vi "Weibull Moments.vi"(9 "b":dbl=3.0, 10 "a":dbl=1.0) -> (0 "error":i32, 2 "variance":dbl=1.0, 3 "mean":dbl)   [LabVIEW 2020, in "NI_Gmath.lvlib"]
doc: "Returns the expected mean and variance of the random variate X, where X describes the selected distribution type. You must manually select the polymorphic instance to use."
uses:
  <vilib>/gmath/NI_Gmath.lvlib
  <vilib>/gmath/statdist.llb/st_error_code.ctl
  <vilib>/gmath/SpecialFunctions.llb/Gamma Function.vi
panel:
  # "Weibull Moments"
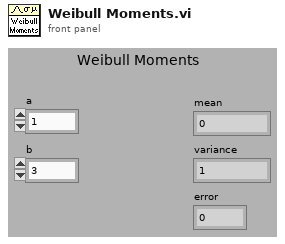
[diagram p1: front panel]
types:
  T1 = typedef "NI_Gmath.lvlib/st_error_code.ctl" = i32
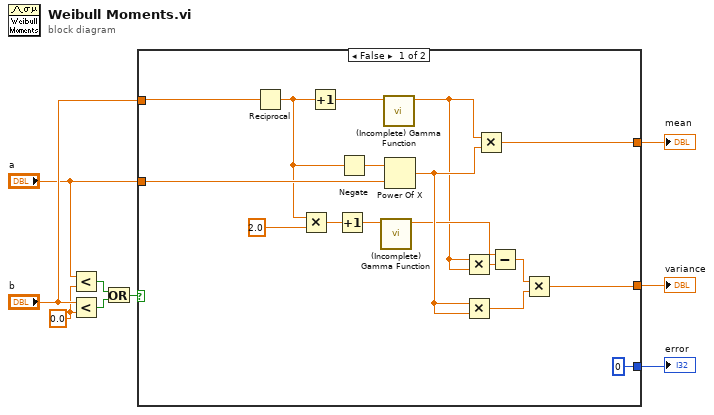
[diagram p0: block diagram]
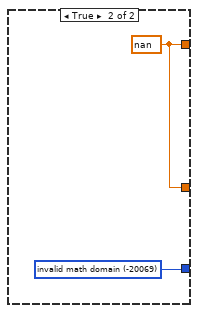
[diagram p2: hidden frame]
diagram:
  w6 = 0.0 ("y")
  n1 = Less?(x="a", y=w6) -> (x < y?=w2:bool)
  n2 = Less?(x="b", y=w6) -> (x < y?=w3:bool)
  n3 = Or(x=w2, y=w3) -> (x .or. y?=w4:bool)
  n4 = case shown="False" w4 {
    tunnel: "b" -> [w25 _]
    tunnel: [0 ("invalid math domain") w27] -> w9
    tunnel: [w22 w28] -> w8
    tunnel: "a" -> [w24 _]
    tunnel: [w15 w28] -> w1
    frame False {
      n5 = Reciprocal(x=w25) -> (1/x=w10:dbl)
      n6 = Multiply(x=w10, y=2.0) -> (x*y=w20:dbl)
      n7 = Increment(x=w10) -> (x+1=w12:dbl)
      n8 = Increment(x=w20) -> (x+1=w14:dbl)
      n9 = Negate(x=w10) -> (-x=w23:dbl)
      n10 = call-poly <vilib>:"(Incomplete) Gamma Function.vi"("x"=w14) -> ("g(x)"=w13:dbl)  [unwired: 10 in]
      n11 = call-poly <vilib>:"(Incomplete) Gamma Function.vi"("x"=w12) -> ("g(x)"=w11:dbl)  [unwired: 10 in]
      n12 = Power Of X(1:w24, 2:w23) -> (0:w18:dbl)
      n13 = Multiply(x=w11, y=w11) -> (x*y=w19:dbl)
      n14 = Multiply(x=w18, y=w18) -> (x*y=w16:dbl)
      n15 = Multiply(x=w11, y=w18) -> (x*y=w22:dbl)
      n16 = Subtract(x=w13, y=w19) -> (x-y=w17:dbl)
      n17 = Multiply(x=w17, y=w16) -> (x*y=w15:dbl)
    }
    frame True {
      w27 = T1 -20069 items=["invalid math domain"=-20069, "Fourier interpolation size m >= n"=-20070, "empty array"=-20003] ("stat interp error code")
      w28 = nan
    }
  }
  "mean" <- w8
  "error" <- w9
  "variance" <- w1
